vi "Configure Panel.vi"(7 "Console Log in":refnum<class "Console Log.lvclass">, 8 "error in":errorcluster, 11 "Gluing Procedure in":refnum<class "Gluing Procedure.lvclass">) -> (0 "error out":errorcluster, 1 "Cancel Button status":bool, 3 "Gluing Procedure out":refnum<class "Gluing Procedure.lvclass">, 5 "Console Log out":refnum<class "Console Log.lvclass">)   [LabVIEW 2011]
uses:
  UI typedefs/Glue Chuck Control.ctl
  UI typedefs/Glue Slot Control.ctl
  UI typedefs/Stamp Chuck Control.ctl
  UI typedefs/Stamp Slot Control.ctl
  Shared Components/Config Manager Class/Type Definitions/Stamp Type.ctl
  UI typedefs/BBM Chuck Used.ctl
  UI typedefs/Weight Chuck Control.ctl
  UI typedefs/Weight Slot Control.ctl
  Shared Components/Config Manager Class/Type Definitions/Weight Type.ctl
  UI typedefs/BM Chuck Control.ctl
  UI typedefs/BM Slot Control.ctl
  UI typedefs/HDI Chuck Control.ctl
  UI typedefs/HDI Slot Control.ctl
  UI typedefs/Glue Paths.ctl
  UI typedefs/Glue Path.ctl
  Procedure Classes/Gluing Procedure/Gluing Procedure.lvclass
  Application Utilities/Console Log/Console Log.lvclass
  UI typedefs/Glue Paths Disable.ctl
  UI typedefs/Active Paths.ctl
  Shared Components/WorkTable Class/WorkTable Class.lvclass
  Procedure Classes/Gluing Procedure/Type Definitions/Configure.ctl
panel:
  out "Active Paths":T1=[TRUE, TRUE, TRUE, TRUE]
  in  "Set all OFF":bool
  in  "Set all ON":bool
  in  "Glue Pathways":T2=[{"HDI Slot "=0, "Stamp Slot"=0, "Glue Slot"=0, "Weight Slot"=0, "BBM Slot"=0}, {"HDI Slot "=1, "Stamp Slot"=1, "Glue Slot"=1, "Weight Slot"=1, "BBM Slot"=1}, {"HDI Slot "=2, "Stamp Slot"=2, "Glue Slot"=2, "Weight Slot"=2, "BBM Slot"=2}, {"HDI Slot "=3, "Stamp Slot"=3, "Glue Slot"=3, "Weight Slot"=3, "BBM Slot"=3}] {"BBM Slot" items=["Slot 1", "Slot 2", "Slot 3", "Slot 4"]; "Weight Slot" items=["Slot 1", "Slot 2", "Slot 3", "Slot 4"]; "Glue Slot" items=["Slot 1", "Slot 2", "Slot 3", "Slot 4"]; "Stamp Slot" items=["Slot 1", "Slot 2", "Slot 3", "Slot 4"]; "HDI Slot" items=["Slot 1", "Slot 2", "Slot 3", "Slot 4"]}
  in  "HDI Chuck Control":T4
  in  "BBM Chuck Control":T6
  in  "Weight Chuck Control":T8={"Slot 1"={"Populated?"=FALSE, "Weight Type"=enum."Weight 1"}, "Slot 2"={"Populated?"=FALSE, "Weight Type"=enum."Weight 2"}, "Slot 3"={"Populated?"=FALSE, "Weight Type"=enum."Weight 3"}, "Slot 4"={"Populated?"=FALSE, "Weight Type"=enum."Weight 4"}}
  in  "Chuck Module Used for BBM:":T11 items=["Chuck 1", "Chuck 2", "Chuck 3", "Chuck 4"]
  in  "Stamp Chuck Control":T12={"Slot 1"={"Populated?"=FALSE, "Stamp Type"=enum."Stamp 1"}, "Slot 2"={"Populated?"=FALSE, "Stamp Type"=enum."Stamp 2"}, "Slot 3"={"Populated?"=FALSE, "Stamp Type"=enum."Stamp 3"}, "Slot 4"={"Populated?"=FALSE, "Stamp Type"=enum."Stamp 4"}}
  in  "Glue Chuck Control":T15
  in  "Cancel Button":bool
  in  "OK Button":bool
  in  "Path Enabling":T17={"Path 1 BG Color"=65280, "Path 2 BG Color"=65280, "Path 3 BG Color"=65280, "Path 4 BG Color"=65280, "Disable Path 1"=FALSE, "Disable Path 2"=FALSE, "Disable Path 3"=FALSE, "Disable Path 4"=FALSE}
  # "Choose your pathways:"
  # "Procedure:\n1.  Select Chucks that are populated\n2.  Use drop down or text box for identification of element.\n3.  Choose path, as needed."
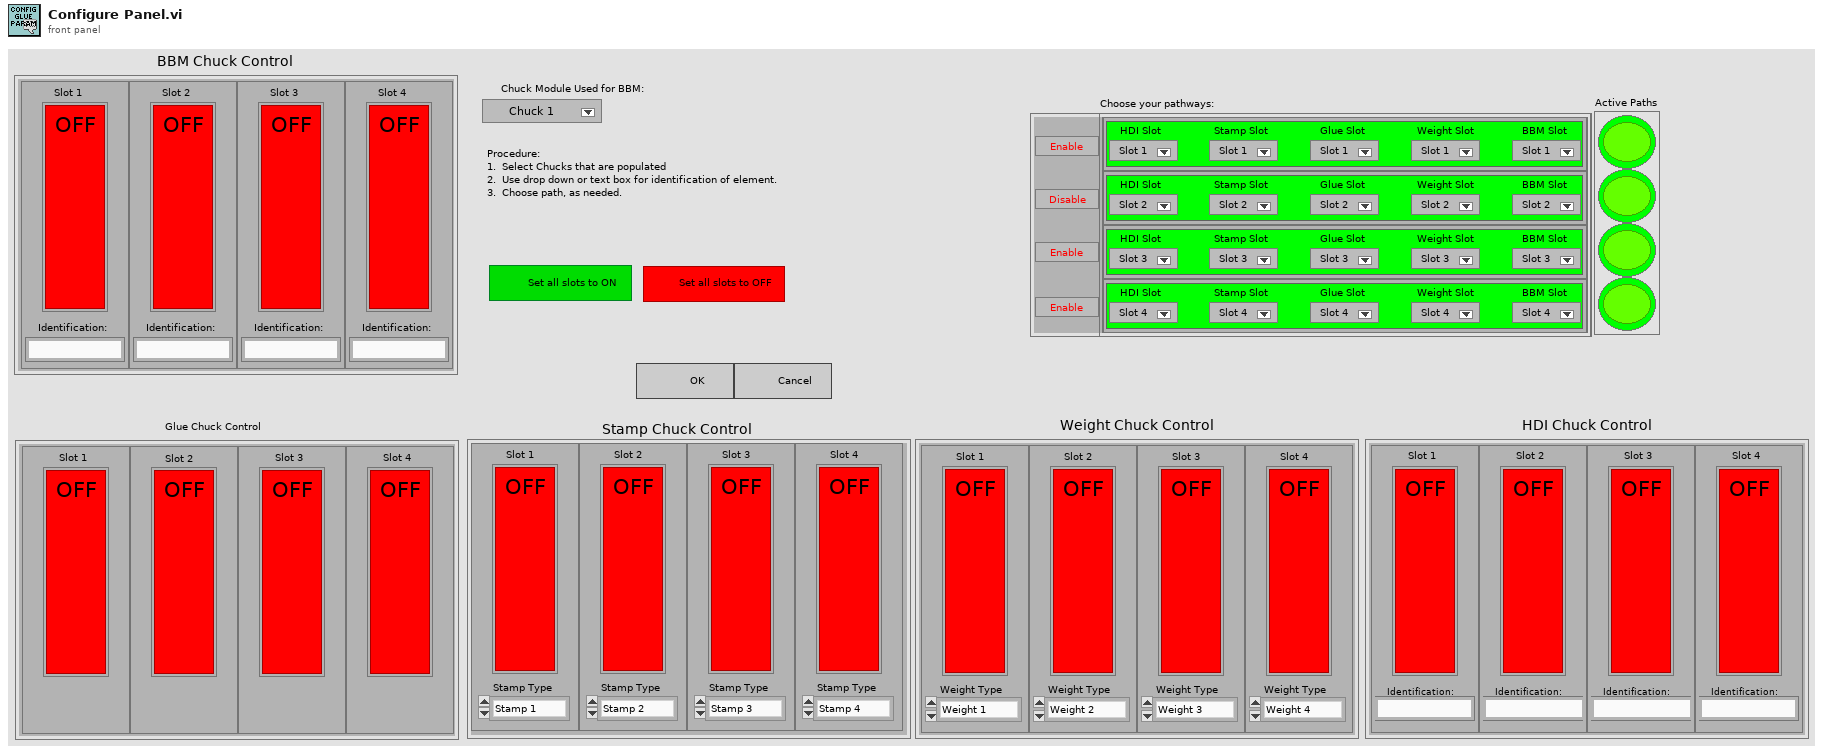
[diagram p1: front panel]
types:
  T1 = typedef "Active Paths.ctl" = bool[]
  T2 = typedef "Glue Paths.ctl" = T3[]
  T3 = typedef "Glue Path.ctl" = cluster{"HDI Slot ":i32, "Stamp Slot":i32, "Glue Slot":i32, "Weight Slot":i32, "BBM Slot":i32}
  T4 = typedef "HDI Chuck Control.ctl" = cluster{"Slot 1":T5, "Slot 2":T5, "Slot 3":T5, "Slot 4":T5}
  T5 = typedef "HDI Slot Control.ctl" = cluster{"Populated?":bool, "Identification:":string}
  T6 = typedef "BM Chuck Control.ctl" = cluster{"Slot 1":T7, "Slot 2":T7, "Slot 3":T7, "Slot 4":T7}
  T7 = typedef "BM Slot Control.ctl" = cluster{"Populated?":bool, "Identification:":string}
  T8 = typedef "Weight Chuck Control.ctl" = cluster{"Slot 1":T9, "Slot 2":T9, "Slot 3":T9, "Slot 4":T9}
  T9 = typedef "Weight Slot Control.ctl" = cluster{"Populated?":bool, "Weight Type":T10}
  T10 = typedef "Weight Type.ctl" = enum16{"Weight 1", "Weight 2", "Weight 3", "Weight 4", "Weight 5", "Weight 6", "Weight 7", "Weight 8"}
  T11 = typedef "BBM Chuck Used.ctl" = i32
  T12 = typedef "Stamp Chuck Control.ctl" = cluster{"Slot 1":T13, "Slot 2":T13, "Slot 3":T13, "Slot 4":T13}
  T13 = typedef "Stamp Slot Control.ctl" = cluster{"Populated?":bool, "Stamp Type":T14}
  T14 = typedef "Stamp Type.ctl" = enum16{"Stamp 1", "Stamp 2", "Stamp 3", "Stamp 4", "Stamp 5"}
  T15 = typedef "Glue Chuck Control.ctl" = cluster{"Slot 1":T16, "Slot 2":T16, "Slot 3":T16, "Slot 4":T16}
  T16 = typedef "Glue Slot Control.ctl" = cluster{"Populated?":bool}
  T17 = typedef "Glue Paths Disable.ctl" = cluster{"Path 1 BG Color":u32, "Path 2 BG Color":u32, "Path 3 BG Color":u32, "Path 4 BG Color":u32, "Disable Path 1":bool, "Disable Path 2":bool, "Disable Path 3":bool, "Disable Path 4":bool}
  T18 = enum16{"Empty", "Bare HDI", "Unglued", "Stamped", "PartOnTop", "Weighted", "Unpotted", "Potted"}
  T19 = typedef "Worktable_Weight.ctl" = cluster{"Weight State":enum16{"Empty", "Populated"}, "Weight Type":T10, "Location/Orientation":T20}
  T20 = typedef "Position_Orientation.ctl" = cluster{"Center":refnum<class "Vec3d Class.lvclass">, "Orientation":refnum<class "Orient3d Class.lvclass">}
  T21 = cluster{"Reservoir State":enum16{"Empty", "Full", "Used"}, "Center":refnum<class "Vec3d Class.lvclass">}
  T22 = typedef "Worktable_Stamp.ctl" = cluster{"Stamp State":enum16{"Empty", "Populated", "Used"}, "Location/Orientation":T20, "Stamp Type":T14}
  T23 = typedef "Worktable_Module Slot.ctl" = cluster{"Slot State":enum16{"Empty", "Bare HDI", "Unglued", "Stamped", "PartOnTop", "Weighted", "Unpotted", "Potted"}, "BBM Type":enum16{"None", "BBM", "GlassSlide"}, "HDI Type":enum16{"None", "HDI", "Polyimide"}, "Vacuum Channel":u8, "Location/Orientation BBM":T20, "Location/Orientation HDI":T20, "S/N":string}
  T24 = cluster{"HDI Chuck Control":refnum<vi>, "Stamp Chuck Control":refnum<vi>, "Glue Chuck Control":refnum<vi>, "Weight Chuck Control":refnum<vi>, "BBM Chuck Control":refnum<vi>}
  T25 = typedef "Configure.ctl" = cluster{"Has been run?":bool, "Active Paths":T1, "Glue Pathways":T2, "Chuck Module Used for BBM:":T11}
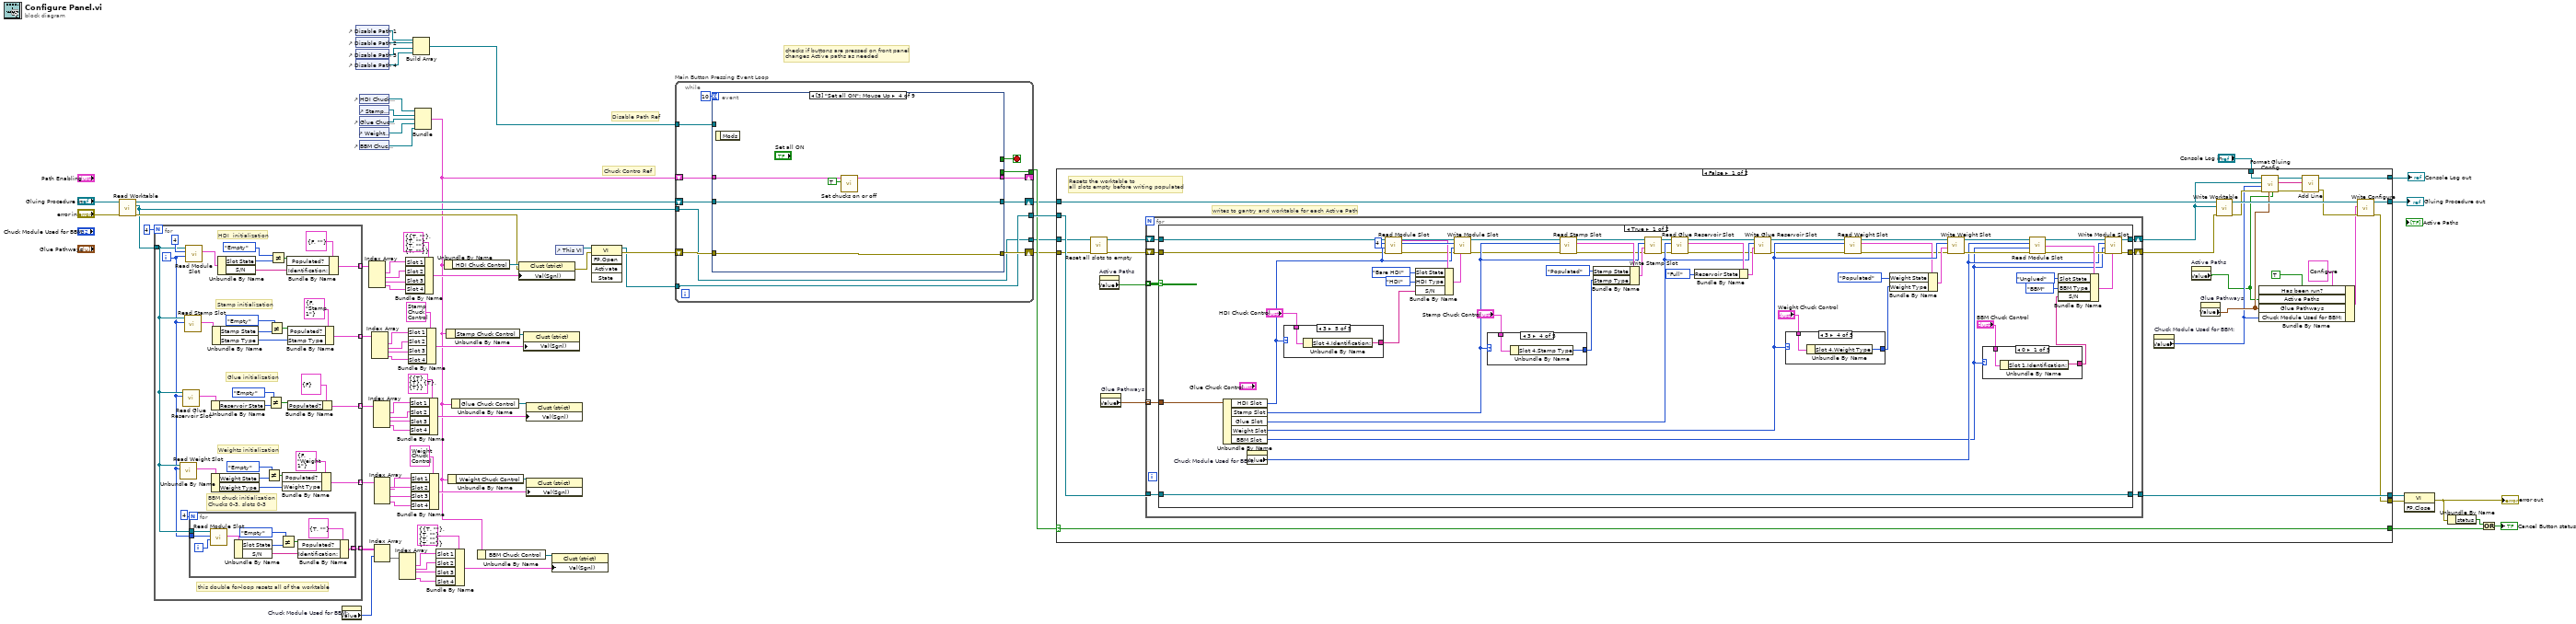
[diagram p0: block diagram]
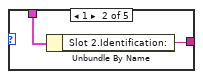
[diagram p2: hidden frame]
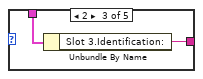
[diagram p3: hidden frame]
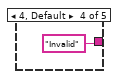
[diagram p4: hidden frame]
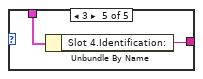
[diagram p5: hidden frame]
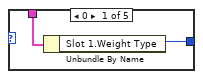
[diagram p6: hidden frame]
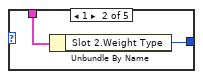
[diagram p7: hidden frame]
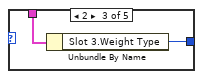
[diagram p8: hidden frame]
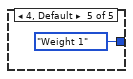
[diagram p9: hidden frame]
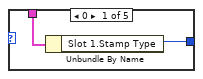
[diagram p10: hidden frame]
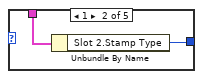
[diagram p11: hidden frame]
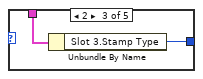
[diagram p12: hidden frame]
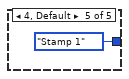
[diagram p13: hidden frame]
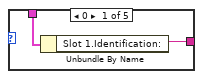
[diagram p14: hidden frame]
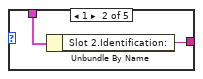
[diagram p15: hidden frame]
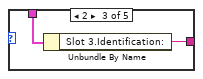
[diagram p16: hidden frame]
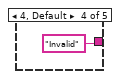
[diagram p17: hidden frame]
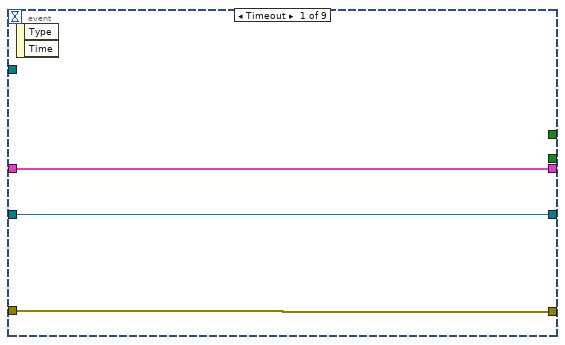
[diagram p20: hidden frame]
diagram:
  # "Chuck Contro Ref"
  # "Disable Path Ref"
  # "checks if buttons are pressed on front panel\nchanges Active paths as needed"
  n1 = call "Read Worktable.vi"("error in"="error in", "Gluing Procedure in"="Gluing Procedure in") -> ("error out"=w10:errorcluster, "WorkTable out"=w7:refnum<class "WorkTable Class.lvclass">, "Gluing Procedure out"=w33:refnum<class "Gluing Procedure.lvclass">)  [unwired: 7 in]
  n2 = for {
    N: 4 -> [_]
    tunnel: [w102] -> w70 mode=indexing
    tunnel: w7 -> [w82]
    tunnel: [w96] -> w13 mode=indexing
    tunnel: [w90] -> w12 mode=indexing
    tunnel: [w84] -> w11 mode=indexing
    tunnel: [w81] -> w3 mode=indexing
    i -> [w80]
    # "this double for-loop resets all of the worktable"
    # "BBM chuck initialization\nChucks 0-3, slots 0-3"
    # "Weights initialization"
    # "Glue initialization"
    # "HDI  initialization"
    # "Stamp initialization"
    n3 = call "Read Weight Slot.vi"("weight slot"=w80, "WorkTable Class in"=w82) -> ("Weight Slot"=w85:T19)  [unwired: 7 in, 2 out]
    n4 = call "Read Glue Reservoir Slot.vi"("index"=w80, "WorkTable Class in"=w82) -> ("Glue Resivoir Slot"=w91:T21)  [unwired: 7 in, 2 out]
    n5 = call "Read Stamp Slot.vi"("Stamp Slot"=w80, "WorkTable Class in"=w82) -> ("Stamp Slot"=w97:T22)  [unwired: 7 in, 2 out]
    n6 = call-dynamic "Read Module Slot.vi"("slot"=w80, "chuck"=4, "WorkTable in"=w82) -> ("Module Slot"=w109:T23)  [unwired: 6 in, 2 out]
    n7 = for {
      N: 4 -> [_]
      tunnel: w82 -> [w116]
      tunnel: [w115] -> w81 mode=indexing
      tunnel: w80 -> [w111]
      i -> [w112]
      n8 = call-dynamic "Read Module Slot.vi"("slot"=w112, "chuck"=w111, "WorkTable in"=w116) -> ("Module Slot"=w119:T23)  [unwired: 6 in, 2 out]
      n9 = Unbundle By Name(w119) -> ("Slot State"=w118:T18, "S/N"=w110:string)
      n10 = Not Equal?(x=T18."Empty", y=w118) -> (x != y?=w117:bool)
      n11 = Bundle By Name(cluster=T7 {"Populated?"=TRUE, "Identification:"=""} ("BBM Slot"), "Populated?"=w117, "Identification:"=w110) -> (w115:T7)
    }
    n12 = Unbundle By Name(w85) -> ("Weight State"=w86:enum16{"Empty", "Populated"}, "Weight Type"=w79:T10)
    n13 = Unbundle By Name(w91) -> ("Reservoir State"=w92:enum16{"Empty", "Full", "Used"})
    n14 = Unbundle By Name(w97) -> ("Stamp State"=w98:enum16{"Empty", "Populated", "Used"}, "Stamp Type"=w78:T14)
    n15 = Unbundle By Name(w109) -> ("Slot State"=w108:T18, "S/N"=w103:string)
    n16 = Not Equal?(x=enum16{"Empty", "Populated"}."Empty", y=w86) -> (x != y?=w87:bool)
    n17 = Not Equal?(x=enum16{"Empty", "Full", "Used"}."Empty", y=w92) -> (x != y?=w93:bool)
    n18 = Not Equal?(x=enum16{"Empty", "Populated", "Used"}."Empty", y=w98) -> (x != y?=w99:bool)
    n19 = Not Equal?(x=T18."Empty", y=w108) -> (x != y?=w105:bool)
    n20 = Bundle By Name(cluster=T9 {"Populated?"=FALSE, "Weight Type"=enum."Weight 1"} ("Weight Slot"), "Populated?"=w87, "Weight Type"=w79) -> (w84:T9)
    n21 = Bundle By Name(cluster=T5 {"Populated?"=FALSE, "Identification:"=""} ("Chuck"), "Populated?"=w105, "Identification:"=w103) -> (w102:T5)
    n22 = Bundle By Name(cluster=T13 {"Populated?"=FALSE, "Stamp Type"=enum."Stamp 1"} ("Stamp Slot"), "Populated?"=w99, "Stamp Type"=w78) -> (w96:T13)
    n23 = Bundle By Name(cluster=T16 {"Populated?"=FALSE} ("Glue Slot"), "Populated?"=w93) -> (w90:T16)
  }
  n24 = property on="Chuck Module Used for BBM:" class="Ring (strict)"() -> ("Value"=w1:i32)  [unwired: 2 in, 2 out]
  n25 = control-ref of="Disable Path 1"() -> (w18:refnum<vi>)
  n26 = control-ref of="Disable Path 2"() -> (w17:refnum<vi>)
  n27 = control-ref of="Disable Path 3"() -> (w16:refnum<vi>)
  n28 = control-ref of="Disable Path 4"() -> (w15:refnum<vi>)
  n29 = control-ref of="BBM Chuck Control"() -> (w5:refnum<vi>)
  n30 = control-ref of="HDI Chuck Control"() -> (w76:refnum<vi>)
  n31 = control-ref of="Stamp Chuck Control"() -> (w75:refnum<vi>)
  n32 = control-ref of="Glue Chuck Control"() -> (w74:refnum<vi>)
  n33 = control-ref of="Weight Chuck Control"() -> (w73:refnum<vi>)
  n34 = Index Array(array=w70) -> (element #1=w68:T5, element #2=w67:T5, element #3=w66:T5, element #4=w65:T5)  [unwired: 4 in]
  n35 = Index Array(array=w13) -> (element #1=w59:T13, element #2=w60:T13, element #3=w61:T13, element #4=w62:T13)  [unwired: 4 in]
  n36 = Index Array(array=w12) -> (element #1=w53:T16, element #2=w52:T16, element #3=w51:T16, element #4=w50:T16)  [unwired: 4 in]
  n37 = Index Array(array=w11) -> (element #1=w42:T9, element #2=w43:T9, element #3=w44:T9, element #4=w45:T9)  [unwired: 4 in]
  n38 = Index Array(array=w3, index (row)=w1) -> (element=w2:T7[])  [unwired: 1 in]
  n39 = Index Array(array=w2) -> (element #1=w40:T7, element #2=w39:T7, element #3=w38:T7, element #4=w37:T7)  [unwired: 4 in]
  n40 = Bundle By Name(cluster=T4 {"Slot 1"={"Populated?"=TRUE, "Identification:"=""}, "Slot 2"={"Populated?"=TRUE, "Identification:"=""}, "Slot 3"={"Populated?"=TRUE, "Identification:"=""}, "Slot 4"={"Populated?"=TRUE, "Identification:"=""}} ("HDI Chuck Control"), "Slot 1"=w68, "Slot 2"=w67, "Slot 3"=w66, "Slot 4"=w65) -> (w63:T4)
  n41 = Bundle By Name(cluster=T12 {"Slot 1"={"Populated?"=TRUE, "Stamp Type"=enum."Stamp 1"}, "Slot 2"={"Populated?"=TRUE, "Stamp Type"=enum."Stamp 2"}, "Slot 3"={"Populated?"=TRUE, "Stamp Type"=enum."Stamp 3"}, "Slot 4"={"Populated?"=TRUE, "Stamp Type"=enum."Stamp 4"}} ("Stamp Chuck Control"), "Slot 1"=w59, "Slot 2"=w60, "Slot 3"=w61, "Slot 4"=w62) -> (w56:T12)
  n42 = Bundle By Name(cluster=T15 {"Slot 1"={"Populated?"=TRUE}, "Slot 2"={"Populated?"=TRUE}, "Slot 3"={"Populated?"=TRUE}, "Slot 4"={"Populated?"=TRUE}} ("Glue Chuck Control"), "Slot 1"=w53, "Slot 2"=w52, "Slot 3"=w51, "Slot 4"=w50) -> (w48:T15)
  n43 = Bundle By Name(cluster=T8 {"Slot 1"={"Populated?"=TRUE, "Weight Type"=enum."Weight 1"}, "Slot 2"={"Populated?"=TRUE, "Weight Type"=enum."Weight 2"}, "Slot 3"={"Populated?"=TRUE, "Weight Type"=enum."Weight 3"}, "Slot 4"={"Populated?"=TRUE, "Weight Type"=enum."Weight 4"}} ("Weight Chuck Control"), "Slot 1"=w42, "Slot 2"=w43, "Slot 3"=w44, "Slot 4"=w45) -> (w47:T8)
  n44 = Build Array(w18, w17, w16, w15) -> (w14:refnum<vi>[])
  n45 = Bundle("HDI Chuck Control"=w76, "Stamp Chuck Control"=w75, "Glue Chuck Control"=w74, "Weight Chuck Control"=w73, "BBM Chuck Control"=w5) -> (w4:T24)  [unwired: 1 in]
  n46 = Bundle By Name(cluster=T6 {"Slot 1"={"Populated?"=TRUE, "Identification:"=""}, "Slot 2"={"Populated?"=TRUE, "Identification:"=""}, "Slot 3"={"Populated?"=TRUE, "Identification:"=""}, "Slot 4"={"Populated?"=TRUE, "Identification:"=""}} ("BM Chuck Control"), "Slot 1"=w40, "Slot 2"=w39, "Slot 3"=w38, "Slot 4"=w37) -> (w35:T6)
  n47 = Unbundle By Name(w4) -> ("HDI Chuck Control"=w64:refnum<vi>)
  n48 = Unbundle By Name(w4) -> ("Stamp Chuck Control"=w57:refnum<vi>)
  n49 = Unbundle By Name(w4) -> ("Weight Chuck Control"=w46:refnum<vi>)
  n50 = Unbundle By Name(w4) -> ("Glue Chuck Control"=w49:refnum<vi>)
  n51 = Unbundle By Name(w4) -> ("BBM Chuck Control"=w36:refnum<vi>)
  n52 = property class="Clust (strict)"(reference=w64, error in=w10, "Val(Sgnl)"=w63) -> (error out=w9:errorcluster)  [unwired: 1 out]
  n53 = property class="Clust (strict)"(reference=w57, "Val(Sgnl)"=w56) -> ()  [unwired: 1 in, 2 out]
  n54 = property class="Clust (strict)"(reference=w49, "Val(Sgnl)"=w48) -> ()  [unwired: 1 in, 2 out]
  n55 = property class="Clust (strict)"(reference=w46, "Val(Sgnl)"=w47) -> ()  [unwired: 1 in, 2 out]
  n56 = property class="Clust (strict)"(reference=w36, "Val(Sgnl)"=w35) -> ()  [unwired: 1 in, 2 out]
  n57 = control-ref of="This VI"() -> (w77:refnum<vi>)
  n58 = invoke class="VI" method="FP.Open"(reference=w77, error in=w9) -> (reference out=w8:refnum<vi>, error out=w32:errorcluster)  [unwired: 3 in, 3 out]
  n59 = while "Main Button Pressing Event Loop" {
    tunnel: [w122] -> w31
    shift-right: [w128] -> w26
    shift-left: w32 -> [w129]
    shift-right: [w126] -> w28
    shift-left: w33 -> [w127]
    tunnel: [w124] -> w29
    tunnel: w14 -> [w123]
    shift-right: [w120] -> _
    shift-left: w4 -> [w130]
    tunnel: w8 -> [w122]
    tunnel: w7 -> [w121]
    tunnel: [w121] -> w6
    stop <- w125 stop-if-true
    n60 = event shown="[3] \"Set all ON\": Mouse Up" {
      selector: _ -> [_ _ _ _ _ _ _ _ _]
      dyn-events: _ -> [_ _ _ _ _ _ _ _ _]
      timeout: 10 -> [_ _ _ _ _ _ _ _ _]
      tunnel: [_ w139 w146 _ _ _ _ _ _] -> w125
      tunnel: w130 -> [w132 w135 w145 w149 w158 w159 w165 w171 w211]
      tunnel: w129 -> [w134 w140 w147 w152 w156 w163 w169 w173 w212]
      tunnel: [w134 w140 w147 w152 w156 w163 w169 w173 w212] -> w128
      tunnel: w127 -> [w133 w141 w148 w151 w155 w164 w170 w172 w213]
      tunnel: [w133 w141 w148 w151 w155 w164 w170 w172 w213] -> w126
      tunnel: [_ _ w146 _ _ _ _ _ _] -> w124
      tunnel: w123 -> [_ _ _ _ _ w161 w167 w174 _]
      tunnel: [w132 w135 w145 w150 w154 w159 w165 w171 w211] -> w120
      event Timeout {
        n61 = event-data() -> ()  [unwired: 1 in, 2 out]
      }
      event "OK Button": Value Change {
        n62 = event-data() -> ()  [unwired: 1 in, 5 out]
        n63 = property on="Active Paths" class="Arr (strict)"() -> ("Value"=w138:bool[])  [unwired: 2 in, 2 out]
        n64 = call "Number of Active Paths.vi"("Active Paths"=w138) -> ("Number of Active Paths"=w137:i32)  [unwired: 10 in]
        n65 = Greater Than 0?(x=w137) -> (x > 0?=w136:bool)
        n66 = case shown="True" w136 {
          tunnel: [FALSE TRUE] -> w139
          frame False {
            n67 = One Button Dialog(message="No active paths are\nenabled.  Please choose\nan active path to continue.") -> ()  [unwired: 1 in, 1 out]
          }
          frame True {
          }
        }
      }
      event "Cancel Button": Value Change {
        w146 = TRUE
        n68 = event-data() -> ()  [unwired: 1 in, 5 out]
      }
      event "Set all ON": Mouse Up {
        n69 = event-data() -> ()  [unwired: 1 in, 1 out]
        n70 = call "Set chucks on or off.vi"("Populated on/off"=TRUE, "Chuck Control ref in"=w149) -> ("Chuck Control ref out"=w150:T24)  [unwired: 8 in, 1 out]
      }
      event "Set all OFF": Mouse Up {
        n71 = event-data() -> ()  [unwired: 1 in, 1 out]
        n72 = call "Set chucks on or off.vi"("Populated on/off"=FALSE, "Chuck Control ref in"=w158) -> ("Chuck Control ref out"=w154:T24)  [unwired: 8 in, 1 out]
      }
      event Value Change {
        n73 = event-data() -> ()  [unwired: 1 in, 5 out]
        n74 = property on="Glue Pathways" class="Arr (strict)"() -> ("Value"=w162:T3[])  [unwired: 2 in, 2 out]
        n75 = call "Check Paths.vi"("Path Disabled Ref"=w161, "Cluster Control ref in"=w159, "Glue Pathways"=w162) -> ("Active Paths"=w160:T1)  [unwired: 8 in]
        n76 = property on="Active Paths" class="Arr (strict)"("Value"=w160) -> ()  [unwired: 2 in, 2 out]
      }
      event Value Change {
        n77 = event-data() -> ()  [unwired: 1 in, 5 out]
        n78 = property on="Glue Pathways" class="Arr (strict)"() -> ("Value"=w168:T3[])  [unwired: 2 in, 2 out]
        n79 = call "Check Paths.vi"("Path Disabled Ref"=w167, "Cluster Control ref in"=w165, "Glue Pathways"=w168) -> ("Active Paths"=w166:T1)  [unwired: 8 in]
        n80 = property on="Active Paths" class="Arr (strict)"("Value"=w166) -> ()  [unwired: 2 in, 2 out]
      }
      event Value Change {
        n81 = event-data() -> ("CtlRef"=w175:refnum<vi>, "NewVal"=w176:bool)  [unwired: 1 in, 3 out]
        n82 = case shown="False" w176 {
          tunnel: w175 -> [w179 w196]
          tunnel: w175 -> [w178 w195]
          tunnel: w174 -> [w177 w194]
          frame True {
            n83 = for {
              tunnel: w177 -> [w183] mode=indexing
              tunnel: w178 -> [w184]
              i -> [w181]
              n84 = Equal?(x=w183, y=w184) -> (x = y?=w182:bool)
              n85 = case shown="True" w182 {
                tunnel: w181 -> [_ w185]
                frame False {
                }
                frame True {
                  n86 = call <vilib>:"RGB to Color.vi"("B"=u8 0, "G"=u8 0, "R"=u8 255) -> ("Color"=w189:u32)
                  n87 = case shown="3" w185 {
                    tunnel: w189 -> [w190 w191 w192 w193 _]
                    frame 0 {
                      n88 = property on="Path 1 BG Color" class="ColBox"("Val(Sgnl)"=w190) -> ()  [unwired: 2 in, 2 out]
                    }
                    frame 1 {
                      n89 = property on="Path 2 BG Color" class="ColBox"("Val(Sgnl)"=w191) -> ()  [unwired: 2 in, 2 out]
                    }
                    frame 2 {
                      n90 = property on="Path 3 BG Color" class="ColBox"("Val(Sgnl)"=w192) -> ()  [unwired: 2 in, 2 out]
                    }
                    frame 3 {
                      n91 = property on="Path 4 BG Color" class="ColBox"("Val(Sgnl)"=w193) -> ()  [unwired: 2 in, 2 out]
                    }
                    frame 4, Default {
                    }
                  }
                }
              }
            }
            n92 = property class="Bool (strict)"(reference=w179, "BoolText.Text"="Enable" ("Label.Text")) -> ()  [unwired: 1 in, 2 out]
          }
          frame False {
            n93 = for {
              tunnel: w194 -> [w200] mode=indexing
              tunnel: w195 -> [w201]
              i -> [w198]
              n94 = Equal?(x=w200, y=w201) -> (x = y?=w199:bool)
              n95 = case shown="True" w199 {
                tunnel: w198 -> [_ w202]
                frame False {
                }
                frame True {
                  n96 = call <vilib>:"RGB to Color.vi"("B"=u8 0, "G"=u8 255, "R"=u8 0) -> ("Color"=w206:u32)
                  n97 = case shown="3" w202 {
                    tunnel: w206 -> [w207 w208 w209 w210 _]
                    frame 0 {
                      n98 = property on="Path 1 BG Color" class="ColBox"("Val(Sgnl)"=w207) -> ()  [unwired: 2 in, 2 out]
                    }
                    frame 1 {
                      n99 = property on="Path 2 BG Color" class="ColBox"("Val(Sgnl)"=w208) -> ()  [unwired: 2 in, 2 out]
                    }
                    frame 2 {
                      n100 = property on="Path 3 BG Color" class="ColBox"("Val(Sgnl)"=w209) -> ()  [unwired: 2 in, 2 out]
                    }
                    frame 3 {
                      n101 = property on="Path 4 BG Color" class="ColBox"("Val(Sgnl)"=w210) -> ()  [unwired: 2 in, 2 out]
                    }
                    frame 4, Default {
                    }
                  }
                }
              }
            }
            n102 = property class="Bool (strict)"(reference=w196, "BoolText.Text"="Disable" ("Label.Text")) -> ()  [unwired: 1 in, 2 out]
          }
        }
      }
      event Panel Close? {
        # "disables the windows X button"
        n103 = event-data() -> ()  [unwired: 1 in, 3 out]
        n104 = event-data("Discard?"=FALSE) -> ()  [unwired: 1 in, 1 out]
      }
    }
  }
  n105 = case shown="False" w29 {
    selector: w29 -> [w238 w347]
    tunnel: w31 -> [w239 w350]
    tunnel: [w240 w350] -> w30
    tunnel: w28 -> [w221 w349]
    tunnel: [w241 w349] -> w27
    tunnel: w26 -> [w218 w348]
    tunnel: [w238 w347] -> w21
    tunnel: [w237 w348] -> w24
    tunnel: "Console Log in" -> [w236 w346]
    tunnel: [w230 w346] -> w19
    tunnel: w6 -> [w220 _]
    frame False {
      # "writes to gantry and worktable for each Active Path"
      # "Resets the worktable to\nall slots empty before writing populated"
      n106 = call "Reset all slots to empty.vi"("error in"=w218, "WorkTable Class in"=w220) -> ("error out"=w217:errorcluster, "WorkTable Class out"=w219:refnum<class "WorkTable Class.lvclass">)  [unwired: 8 in]
      n107 = property on="Active Paths" class="Arr (strict)"() -> ("Value"=w224:bool[])  [unwired: 2 in, 2 out]
      n108 = property on="Glue Pathways" class="Arr (strict)"() -> ("Value"=w222:T3[])  [unwired: 2 in, 2 out]
      n109 = for {
        tunnel: w224 -> [w250] mode=indexing
        shift-right: [w248] -> w216
        shift-left: w219 -> [w249]
        shift-right: [w247] -> w215
        shift-left: w217 -> [w246]
        tunnel: [w245] -> w240
        tunnel: w239 -> [w244]
        tunnel: w222 -> [w243] mode=indexing
        n110 = case shown="True" w250 {
          tunnel: w249 -> [w306 w344]
          tunnel: [w272 w344] -> w248
          tunnel: [w271 w343] -> w247
          tunnel: w246 -> [w260 w343]
          tunnel: [w259 w345] -> w245
          tunnel: w244 -> [w259 w345]
          tunnel: w243 -> [w254 _]
          frame True {
            w305 = 4 ("chuck")
            n111 = Unbundle By Name(w254) -> ("HDI Slot"=w293:i32, "Stamp Slot"=w292:i32, "Glue Slot"=w286:i32, "Weight Slot"=w283:i32, "BBM Slot"=w252:i32)
            n112 = property on="Chuck Module Used for BBM:" class="Ring (strict)"() -> ("Value"=w255:i32)  [unwired: 2 in, 2 out]
            n113 = case shown="3" w293 {
              tunnel: "HDI Chuck Control" -> [w335 w337 w339 _ w342]
              tunnel: [w334 w336 w338 "Invalid" w341] -> w301
              frame 0 {
                n114 = Unbundle By Name(w335) -> ("Slot 1.Identification:"=w334:string)
              }
              frame 1 {
                n115 = Unbundle By Name(w337) -> ("Slot 2.Identification:"=w336:string)
              }
              frame 2 {
                n116 = Unbundle By Name(w339) -> ("Slot 3.Identification:"=w338:string)
              }
              frame 4, Default {
              }
              frame 3 {
                n117 = Unbundle By Name(w342) -> ("Slot 4.Identification:"=w341:string)
              }
            }
            n118 = call-dynamic "Read Module Slot.vi"("error in"=w260, "slot"=w293, "chuck"=w305, "WorkTable in"=w306) -> ("error out"=w261:errorcluster, "Module Slot"=w304:T23, "WorkTable out"=w300:refnum<class "WorkTable Class.lvclass">)  [unwired: 5 in]
            n119 = Bundle By Name(cluster=w304, "Slot State"=T18."Bare HDI", "HDI Type"=enum16{"None", "HDI", "Polyimide"}."HDI", "S/N"=w301) -> (w262:T23)
            n120 = call-dynamic "Write Module Slot.vi"("Module Slot"=w262, "error in"=w261, "slot"=w293, "chuck"=w305, "WorkTable in"=w300) -> ("error out"=w263:errorcluster, "WorkTable out"=w299:refnum<class "WorkTable Class.lvclass">)  [unwired: 5 in]
            n121 = case shown="3" w292 {
              tunnel: "Stamp Chuck Control" -> [w326 w328 w330 w332 _]
              tunnel: [w325 w327 w329 w331 Stamp_Type."Stamp 1" ("Stamp Type")] -> w294
              frame 0 {
                n122 = Unbundle By Name(w326) -> ("Slot 1.Stamp Type"=w325:T14)
              }
              frame 1 {
                n123 = Unbundle By Name(w328) -> ("Slot 2.Stamp Type"=w327:T14)
              }
              frame 2 {
                n124 = Unbundle By Name(w330) -> ("Slot 3.Stamp Type"=w329:T14)
              }
              frame 3 {
                n125 = Unbundle By Name(w332) -> ("Slot 4.Stamp Type"=w331:T14)
              }
              frame 4, Default {
              }
            }
            n126 = call "Read Stamp Slot.vi"("error in (no error)"=w263, "Stamp Slot"=w292, "WorkTable Class in"=w299) -> ("error out"=w264:errorcluster, "Stamp Slot"=w298:T22, "WorkTable Class out"=w296:refnum<class "WorkTable Class.lvclass">)  [unwired: 6 in]
            n127 = Bundle By Name(cluster=w298, "Stamp State"=enum16{"Empty", "Populated", "Used"}."Populated", "Stamp Type"=w294) -> (w295:T22)
            n128 = call "Write Stamp Slot.vi"("error in (no error)"=w264, 9:"Stamp Slot"=w295, 10:"Stamp Slot"=w292, "WorkTable Class in"=w296) -> ("error out"=w265:errorcluster, "WorkTable Class out"=w291:refnum<class "WorkTable Class.lvclass">)  [unwired: 6 in]
            n129 = call "Read Glue Reservoir Slot.vi"("error in (no error)"=w265, "index"=w286, "WorkTable Class in"=w291) -> ("error out"=w266:errorcluster, "Glue Resivoir Slot"=w290:T21, "WorkTable Class out"=w288:refnum<class "WorkTable Class.lvclass">)  [unwired: 6 in]
            n130 = Bundle By Name(cluster=w290, "Reservoir State"=enum16{"Empty", "Full", "Used"}."Full") -> (w287:T21)
            n131 = call "Write Glue Reservoir Slot.vi"("error in (no error)"=w266, "Glue Resivoir Slot"=w287, "index"=w286, "WorkTable Class in"=w288) -> ("error out"=w267:errorcluster, "WorkTable Class out"=w285:refnum<class "WorkTable Class.lvclass">)  [unwired: 6 in]
            n132 = case shown="3" w283 {
              tunnel: "Weight Chuck Control" -> [w317 w319 w321 w323 _]
              tunnel: [w316 w318 w320 w322 Weight_Type."Weight 1" ("Weight Type")] -> w280
              frame 0 {
                n133 = Unbundle By Name(w317) -> ("Slot 1.Weight Type"=w316:T10)
              }
              frame 1 {
                n134 = Unbundle By Name(w319) -> ("Slot 2.Weight Type"=w318:T10)
              }
              frame 2 {
                n135 = Unbundle By Name(w321) -> ("Slot 3.Weight Type"=w320:T10)
              }
              frame 3 {
                n136 = Unbundle By Name(w323) -> ("Slot 4.Weight Type"=w322:T10)
              }
              frame 4, Default {
              }
            }
            n137 = call "Read Weight Slot.vi"("error in (no error)"=w267, "weight slot"=w283, "WorkTable Class in"=w285) -> ("error out"=w268:errorcluster, "Weight Slot"=w282:T19, "WorkTable Class out"=w284:refnum<class "WorkTable Class.lvclass">)  [unwired: 6 in]
            n138 = Bundle By Name(cluster=w282, "Weight State"=enum16{"Empty", "Populated"}."Populated", "Weight Type"=w280) -> (w279:T19)
            n139 = call "Write Weight Slot.vi"("error in (no error)"=w268, "Weight Slot"=w279, "weight slot"=w283, "WorkTable Class in"=w284) -> ("error out"=w269:errorcluster, "WorkTable Class out"=w275:refnum<class "WorkTable Class.lvclass">)  [unwired: 6 in]
            n140 = case shown="0" w252 {
              tunnel: "BBM Chuck Control" -> [w308 w310 w312 _ w315]
              tunnel: [w307 w309 w311 "Invalid" w314] -> w251
              frame 0 {
                n141 = Unbundle By Name(w308) -> ("Slot 1.Identification:"=w307:string)
              }
              frame 1 {
                n142 = Unbundle By Name(w310) -> ("Slot 2.Identification:"=w309:string)
              }
              frame 2 {
                n143 = Unbundle By Name(w312) -> ("Slot 3.Identification:"=w311:string)
              }
              frame 4, Default {
              }
              frame 3 {
                n144 = Unbundle By Name(w315) -> ("Slot 4.Identification:"=w314:string)
              }
            }
            n145 = call-dynamic "Read Module Slot.vi"("error in"=w269, "slot"=w252, "chuck"=w255, "WorkTable in"=w275) -> ("error out"=w270:errorcluster, "Module Slot"=w276:T23, "WorkTable out"=w278:refnum<class "WorkTable Class.lvclass">)  [unwired: 5 in]
            n146 = Bundle By Name(cluster=w276, "Slot State"=T18."Unglued", "BBM Type"=enum16{"None", "BBM", "GlassSlide"}."BBM", "S/N"=w251) -> (w273:T23)
            n147 = call-dynamic "Write Module Slot.vi"("Module Slot"=w273, "error in"=w270, "slot"=w252, "chuck"=w255, "WorkTable in"=w278) -> ("error out"=w271:errorcluster, "WorkTable out"=w272:refnum<class "WorkTable Class.lvclass">)  [unwired: 5 in]
          }
          frame False {
          }
        }
      }
      n148 = property on="Chuck Module Used for BBM:" class="Ring (strict)"() -> ("Value"=w226:i32)  [unwired: 2 in, 2 out]
      n149 = property on="Active Paths" class="Arr (strict)"() -> ("Value"=w223:bool[])  [unwired: 2 in, 2 out]
      n150 = property on="Glue Pathways" class="Arr (strict)"() -> ("Value"=w227:T3[])  [unwired: 2 in, 2 out]
      n151 = call "Write Worktable.vi"("error in"=w215, "WorkTable"=w216, "Gluing Procedure in"=w221) -> ("error out"=w233:errorcluster, "Gluing Procedure out"=w242:refnum<class "Gluing Procedure.lvclass">)  [unwired: 7 in]
      n152 = Bundle By Name(cluster=T25 {"Has been run?"=FALSE, "Active Paths"=[TRUE, TRUE, TRUE, TRUE], "Glue Pathways"=[{"HDI Slot "=0, "Stamp Slot"=0, "Glue Slot"=0, "Weight Slot"=0, "BBM Slot"=0}, {"HDI Slot "=1, "Stamp Slot"=1, "Glue Slot"=1, "Weight Slot"=1, "BBM Slot"=1}, {"HDI Slot "=2, "Stamp Slot"=2, "Glue Slot"=2, "Weight Slot"=2, "BBM Slot"=2}, {"HDI Slot "=3, "Stamp Slot"=3, "Glue Slot"=3, "Weight Slot"=3, "BBM Slot"=3}], "Chuck Module Used for BBM:"=0} ("Configure"), "Has been run?"=TRUE, "Active Paths"=w223, "Glue Pathways"=w227, "Chuck Module Used for BBM:"=w226) -> (w225:T25)
      n153 = call "Format Gluing Config.vi"("Active Paths"=w223, "Glue Pathways"=w227, "error in"=w233, "Chuck Module Used for BBM:"=w226, "Worktable"=w216, "Console Log in"=w236) -> ("error out"=w232:errorcluster, "Formatted Worktable Config"=w234:string, "Console Log out"=w235:refnum<class "Console Log.lvclass">)  [unwired: 3 in]
      n154 = call "Add Line.vi"("error in"=w232, "String"=w234, "Console Log in"=w235) -> ("error out"=w231:errorcluster, "Console Log out"=w230:refnum<class "Console Log.lvclass">)  [unwired: 7 in]
      n155 = call "Write Configure.vi"("error in (no error)"=w231, "Configure"=w225, "Gluing Procedure in"=w242) -> ("error out"=w237:errorcluster, "Gluing Procedure out"=w241:refnum<class "Gluing Procedure.lvclass">)  [unwired: 7 in]
    }
    frame True {
    }
  }
  "Gluing Procedure out" <- w27
  "Console Log out" <- w19
  n156 = invoke class="VI" method="FP.Close"(reference=w30, error in=w24) -> (error out=w23:errorcluster)  [unwired: 1 in, 2 out]
  "error out" <- w23
  n157 = Unbundle By Name(w23) -> ("status"=w22:bool)
  n158 = Or(x=w22, y=w21) -> (x .or. y?=→"Cancel Button status":bool)
